vi "OnSystemButton.vi"(8 "error in (no error)":errorcluster, 10 "State":T1, 11 "Game in":refnum<class "Game.lvclass">) -> (0 "error out":errorcluster, 3 "Game out":refnum<class "Game.lvclass">)   [LabVIEW 2019, in "RT_Game.lvlib" / "Game.lvclass"]
uses:
  Game.lvclass
  Menu/States.ctl
  Game.lvclass/Game.ctl
  GameMenu/GameMenu.lvclass/GameMenu.ctl
  GameMenu/Read Active_.vi
  GameMenu/GameMenu.lvclass
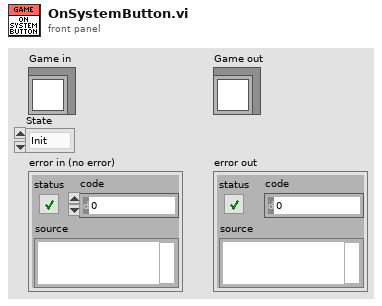
[diagram p1: front panel]
types:
  T1 = typedef "RT_Game.lvlib/Game.lvclass/States.ctl" = enum16{"Init", "Restart", "Menu", "Game", "Resume", "ToggleSingleplayer", "LoadNextGame", "ExitToMenu", "NewHighscore", "GameOver", "SlideOut"}
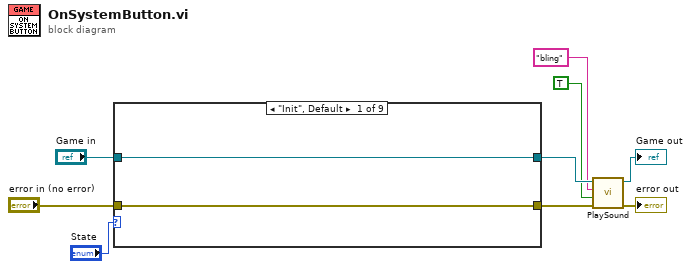
[diagram p0: block diagram]
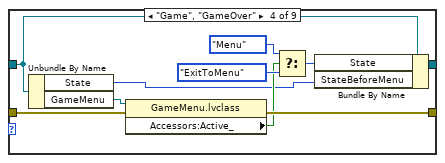
[diagram p4: hidden frame]
diagram:
  n1 = case shown="\"Init\", Default" "State" {
    tunnel: [w10 w12 w14 w25 w26 w28 w30 w32 w34] -> w9
    tunnel: "error in (no error)" -> [w10 w12 w14 w24 w26 w28 w30 w32 w34]
    tunnel: "Game in" -> [w11 w13 w15 w18 w27 w29 w31 w33 w35]
    tunnel: [w11 w13 w15 w17 w27 w29 w31 w33 w35] -> w4
    frame "Init", Default {
    }
    frame "Restart" {
    }
    frame "Menu" {
    }
    frame "Game", "GameOver" {
      n2 = Unbundle By Name(w18) -> ("State"=w16:T1, "GameMenu"=w19:refnum<class "GameMenu.lvclass">)
      n3 = property class="GameMenu.lvclass"(reference=w19, error in=w24) -> (error out=w25:errorcluster, "Accessors:Active_"=w22:bool)  [unwired: 1 out]
      n4 = Select(t=States."Menu" ("State"), s=w22, f=States."ExitToMenu") -> (s? t:f=w20:T1)
      n5 = Bundle By Name(cluster=w18, "State"=w20, "StateBeforeMenu"=w16) -> (w17:refnum<class "Game.lvclass">)
    }
    frame "Resume" {
    }
    frame "ToggleSingleplayer" {
    }
    frame "LoadNextGame" {
    }
    frame "ExitToMenu" {
    }
    frame "SlideOut" {
    }
  }
  n6 = call "PlaySound.vi"("error in (no error)"=w9, "Overwrite"=TRUE, "Name"="bling", "Game in"=w4) -> ("error out"=→"error out":errorcluster, "Game out"=→"Game out":refnum<class "Game.lvclass">)  [unwired: 6 in]
